vi "WPI_CANTalonSRX_Global.vi"(4 "32-bit Frame":u32, 6 "Set Boolean":bool, 7 "Write After Receive":T2, 8 "Set Number":dbl, 9 "Control Mode":T1, 10 "Operation":T7, 11 "Device ID (0)":u8) -> (1 "Get All":T2, 3 "Device ID Out":u8, 5 "Read For Send":T3={"Output"=0.0, "Control Mode"=enum."Percent VBus", "Brake-Mode Override"=enum."No Override", "Reverse Feedback Sensor"=FALSE, "Reverse Closed-Loop Output"=FALSE, "Override Limits"=FALSE, "Forward Limit Enabled"=FALSE, "Reverse Limit Enabled"=FALSE, "Feedback Select"=0, "Profile Select"=0, "Master To Follow"=0, "Throttle Ramp Rate"=0, "Disabled"=FALSE, "Encoder Codes Per Rev"=0, "Num Pot Turns"=0, "Control Frame Rate Ms"=0, "Use Control5 If Supported"=FALSE, "Enable Frame Rate Ms"=10, "Motion Profile Flow Control"=0, "Motion Profile Control Frame Rate"=10, "Talon SRX Motion Profile Trajectory Point"={"Duration Ms"=0, "Velocity"=0.0, "Position"=0.0, "Profile Slot Select"=0, "Is Last"=FALSE, "Velocity Only"=FALSE, "Zero Position"=FALSE, "Compress Code"=0, "Same Velocity"=0, "Delta Position"=0, "Count"=0}, "Current Limit Enabled"=FALSE} {"Feedback Select" items=["Digital Quadrature Encoder"=0, "Analog Pot"=2, "Analog Encoder"=3, "Count on Quad-A (Rising-Edge)"=4, "Count on Quad-A (Falling-Edge)"=5, "Position is Pulse-Width"=8, "CTR Magnetic Enc (Relative)"=6, "CTR Magnetic Enc (Absolute)"=7]})   [LabVIEW 2016]
uses:
  <vilib>/Rock Robotics/WPI/ThirdParty/CanMotor/TalonSRX/WPI_CANTalonSRX_GlobalOps.ctl
  <vilib>/Rock Robotics/WPI/ThirdParty/CanMotor/TalonSRX/WPI_CANTalonSRX_GlobalControl.ctl
  <vilib>/Rock Robotics/WPI/ThirdParty/CanMotor/TalonSRX/WPI_CANTalonSRX_APIControlMode.ctl
  <vilib>/Rock Robotics/WPI/ThirdParty/CanMotor/TalonSRX/WPI_CANTalonSRX_BrakeOverride.ctl
  <vilib>/Rock Robotics/WPI/ThirdParty/CanMotor/TalonSRX/WPI_CANTalonSRX_FeedbackSelect.ctl
  <vilib>/Rock Robotics/WPI/ThirdParty/CanMotor/TalonSRX/WPI_CANTalonSRX_MotionProfileTrajectoryPt.ctl
  <vilib>/Rock Robotics/WPI/ThirdParty/CanMotor/TalonSRX/WPI_CANTalonSRX_GlobalStatus.ctl
  <vilib>/Rock Robotics/WPI/ThirdParty/CanMotor/TalonSRX/WPI_CANTalonSRX_MessageIDs.ctl
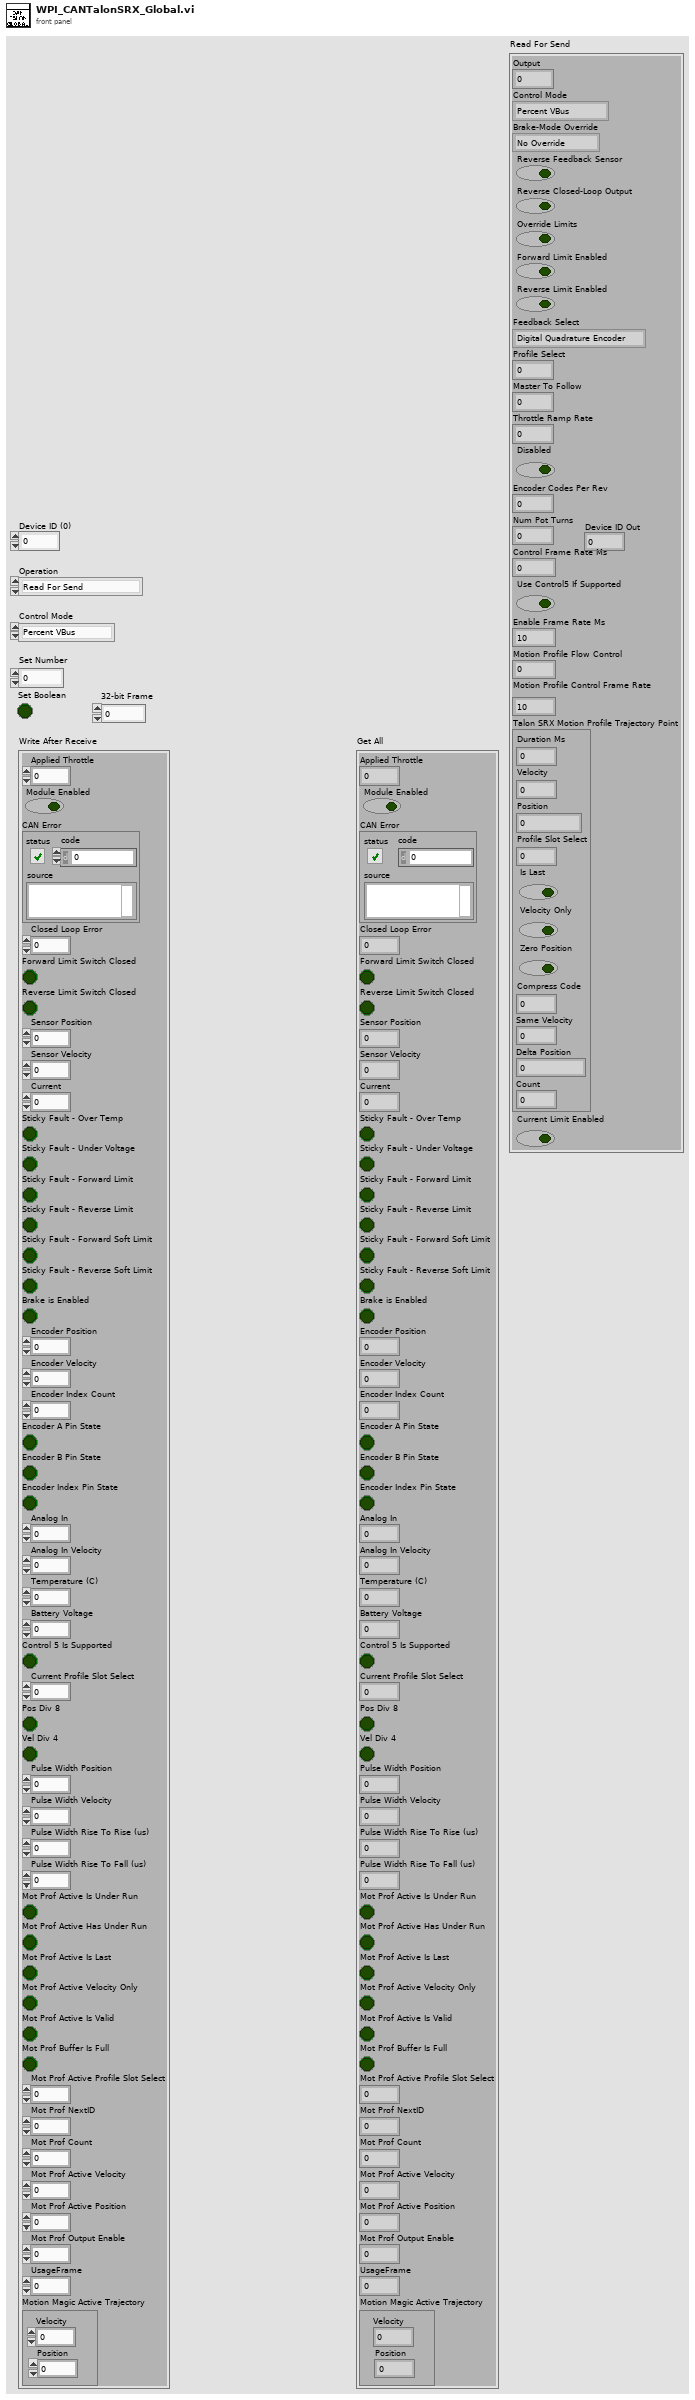
[diagram p1: front panel]
types:
  T1 = typedef "WPI_CANTalonSRX_APIControlMode.ctl" = enum8{"Percent VBus", "Speed", "Position", "Slave", "Unchanged / Invalid", "Voltage Compensation", "Current", "Motion Profile", "Motion Magic"}
  T2 = typedef "WPI_CANTalonSRX_GlobalStatus.ctl" = cluster{"Applied Throttle":dbl, "Module Enabled":bool, "CAN Error":errorcluster, "Closed Loop Error":dbl, "Forward Limit Switch Closed":bool, "Reverse Limit Switch Closed":bool, "Sensor Position":dbl, "Sensor Velocity":dbl, "Current":dbl, "Sticky Fault - Over Temp":bool, "Sticky Fault - Under Voltage":bool, "Sticky Fault - Forward Limit":bool, "Sticky Fault - Reverse Limit":bool, "Sticky Fault - Forward Soft Limit":bool, "Sticky Fault - Reverse Soft Limit":bool, "Brake is Enabled":bool, "Encoder Position":dbl, "Encoder Velocity":dbl, "Encoder Index Count":dbl, "Encoder A Pin State":bool, "Encoder B Pin State":bool, "Encoder Index Pin State":bool, "Analog In":dbl, "Analog In Velocity":dbl, "Temperature (C)":dbl, "Battery Voltage":dbl, "Control 5 Is Supported":bool, "Current Profile Slot Select":dbl, "Pos Div 8":bool, "Vel Div 4":bool, "Pulse Width Position":i32, "Pulse Width Velocity":i32, "Pulse Width Rise To Rise (us)":i32, "Pulse Width Rise To Fall (us)":i32, "Mot Prof Active Is Under Run":bool, "Mot Prof Active Has Under Run":bool, "Mot Prof Active Is Last":bool, "Mot Prof Active Velocity Only":bool, "Mot Prof Active Is Valid":bool, "Mot Prof Buffer Is Full":bool, "Mot Prof Active Profile Slot Select":i32, "Mot Prof NextID":i32, "Mot Prof Count":i32, "Mot Prof Active Velocity":dbl, "Mot Prof Active Position":dbl, "Mot Prof Output Enable":i32, "UsageFrame":u32, "Motion Magic Active Trajectory":cluster{"Velocity":dbl, "Position":dbl}}
  T3 = typedef "WPI_CANTalonSRX_GlobalControl.ctl" = cluster{"Output":dbl, "Control Mode":T1, "Brake-Mode Override":T4, "Reverse Feedback Sensor":bool, "Reverse Closed-Loop Output":bool, "Override Limits":bool, "Forward Limit Enabled":bool, "Reverse Limit Enabled":bool, "Feedback Select":T5, "Profile Select":u8, "Master To Follow":u8, "Throttle Ramp Rate":u8, "Disabled":bool, "Encoder Codes Per Rev":u32, "Num Pot Turns":u32, "Control Frame Rate Ms":u8, "Use Control5 If Supported":bool, "Enable Frame Rate Ms":u8, "Motion Profile Flow Control":u8, "Motion Profile Control Frame Rate":u8, "Talon SRX Motion Profile Trajectory Point":T6, "Current Limit Enabled":bool}
  T4 = typedef "WPI_CANTalonSRX_BrakeOverride.ctl" = enum8{"No Override", "Override to Coast", "Override to Brake"}
  T5 = typedef "WPI_CANTalonSRX_FeedbackSelect.ctl" = u8
  T6 = typedef "WPI_CANTalonSRX_MotionProfileTrajectoryPt.ctl" = cluster{"Duration Ms":u8, "Velocity":dbl, "Position":dbl, "Profile Slot Select":u8, "Is Last":bool, "Velocity Only":bool, "Zero Position":bool, "Compress Code":u8, "Same Velocity":i32, "Delta Position":i32, "Count":u8}
  T7 = typedef "WPI_CANTalonSRX_GlobalOps.ctl" = enum16{"Read For Send", "Write After Receive General", "Write After Receive Feedback", "Write After Receive Encoder", "Write After Receive Ain", "Write Error", "Get All", "Set Output", "Set Mode", "Set Master ID", "Set Brake Mode", "Set Reverse Feedback Sensor", "Set Reverse Closed Loop Output", "Set Override Limits", "Set Forward Limit Enabled", "Set Reverse Limit Enabled", "Set Feedback Select", "Set Profile Select", "Set Throttle Ramp Rate", "Disable", "Set Enc Codes Per Rev", "Set Num Pot Turns", "Set Control Frame Rate", "Enable Legacy Control", "Write After Receive Pulse Width", "Set Enable Frame Rate", "Write After Receive Motion Profile", "Set Motion Profile Flow Control", "Set Motion Profile Control Frame Rate", "Set Current Limit Enable", "Set Usage Frame", "Write After Receive Motion Magic"}
  T8 = typedef "WPI_CANTalonSRX_MessageIDs.ctl" = u32
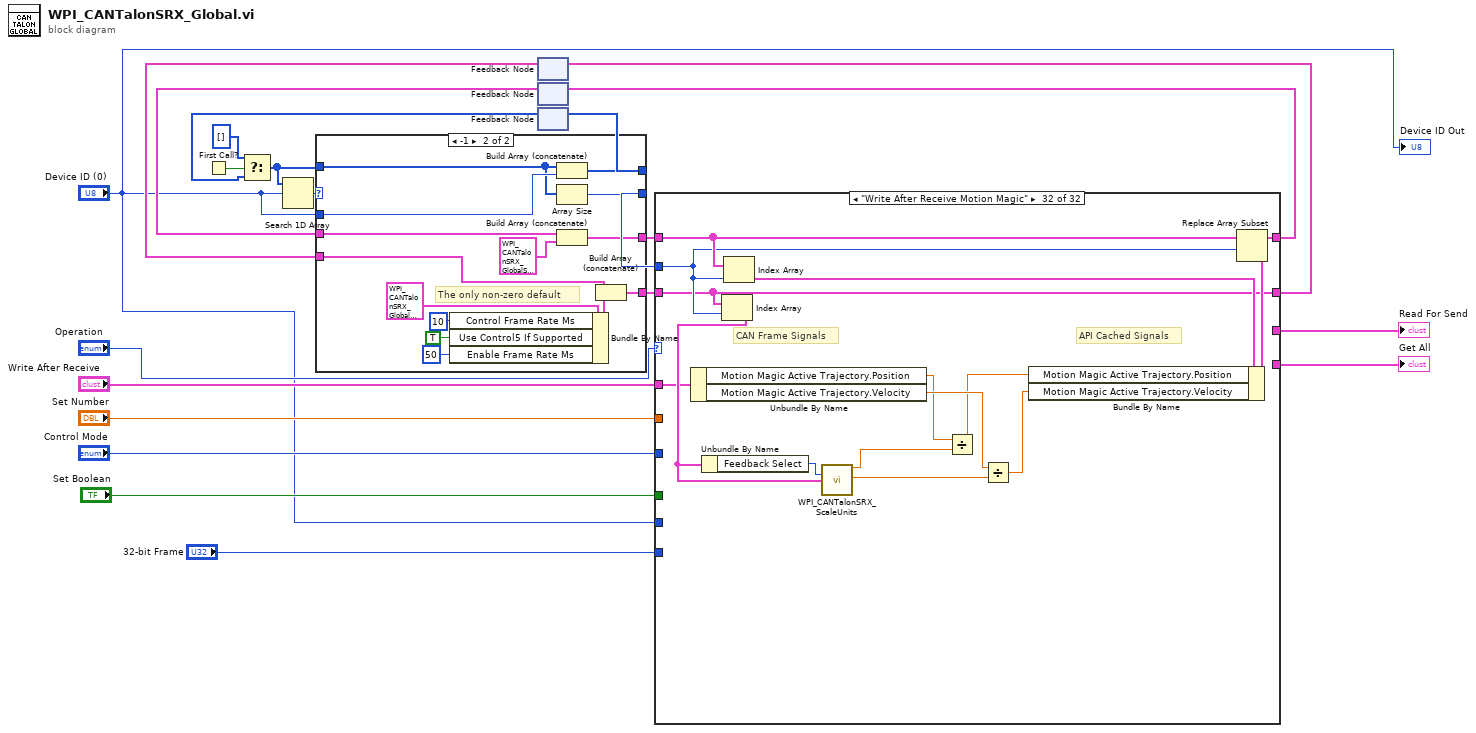
[diagram p0: block diagram]
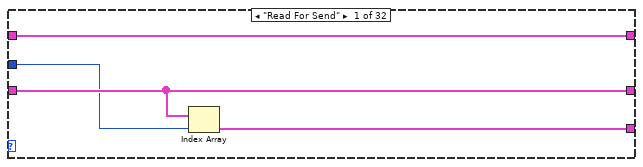
[diagram p2: hidden frame]
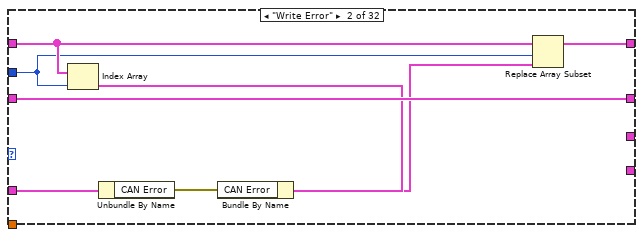
[diagram p3: hidden frame]
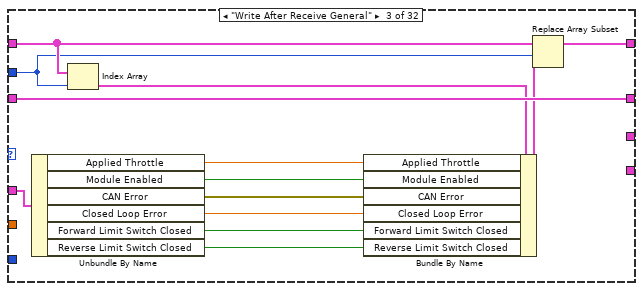
[diagram p4: hidden frame]
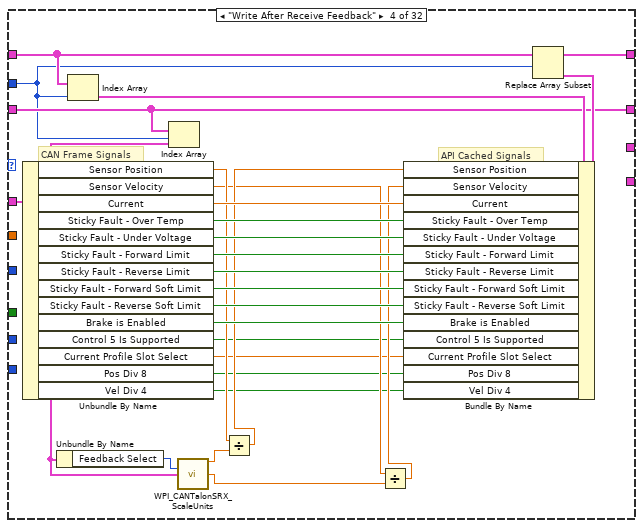
[diagram p5: hidden frame]
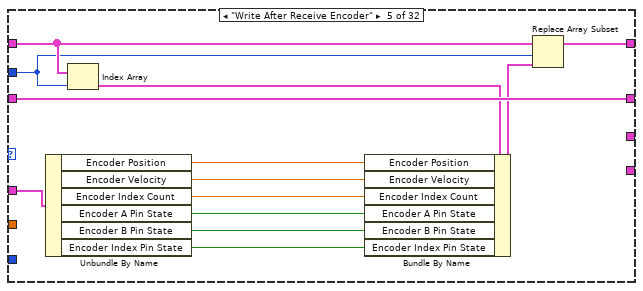
[diagram p6: hidden frame]
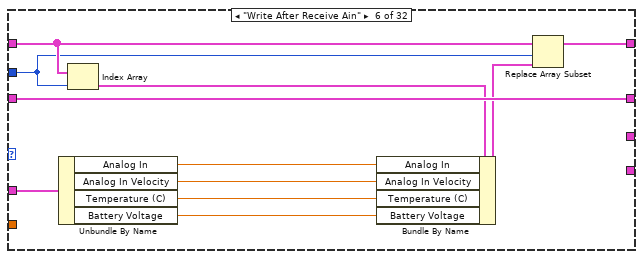
[diagram p7: hidden frame]
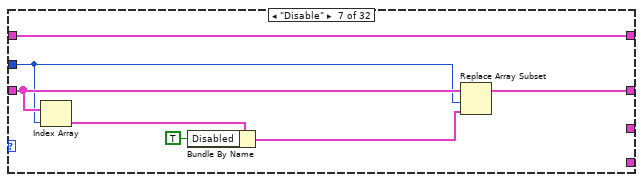
[diagram p8: hidden frame]
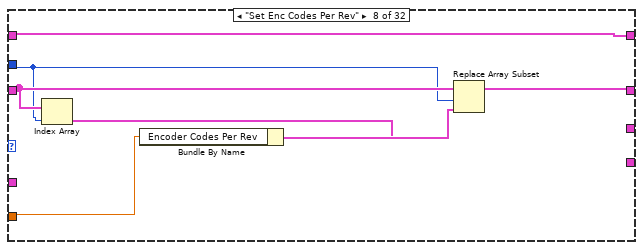
[diagram p9: hidden frame]
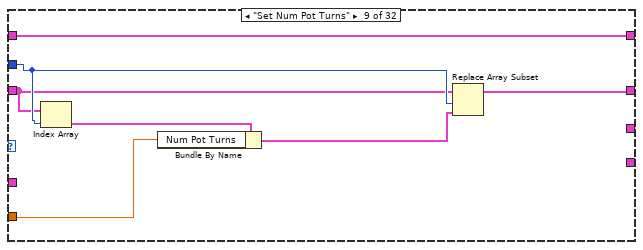
[diagram p10: hidden frame]
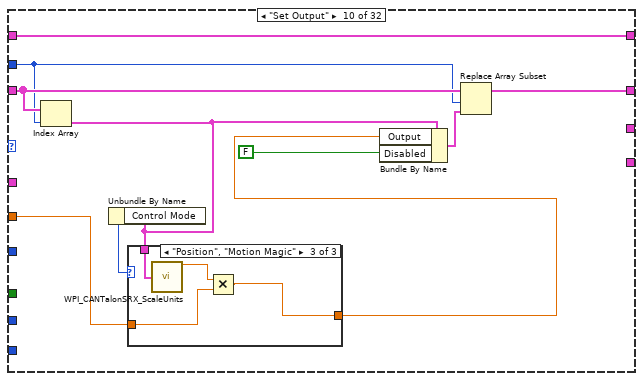
[diagram p11: hidden frame]
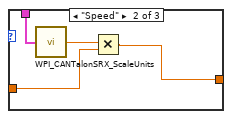
[diagram p13: hidden frame]
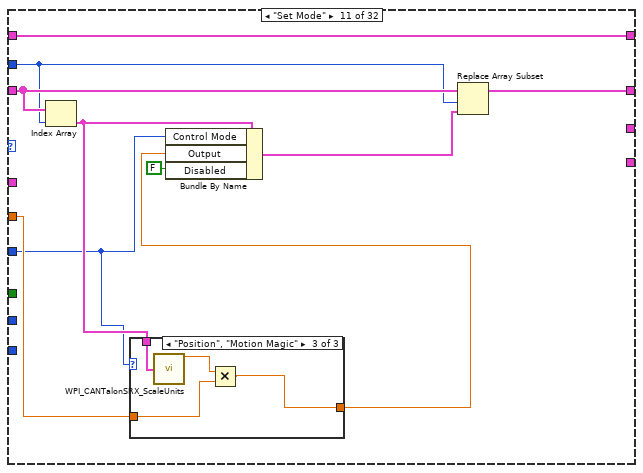
[diagram p14: hidden frame]
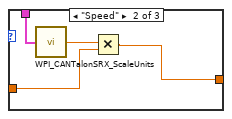
[diagram p16: hidden frame]
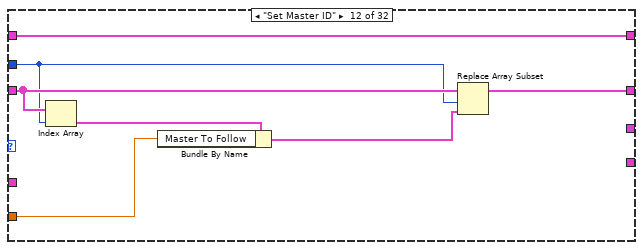
[diagram p17: hidden frame]
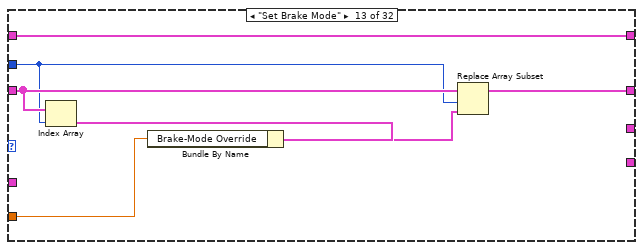
[diagram p18: hidden frame]
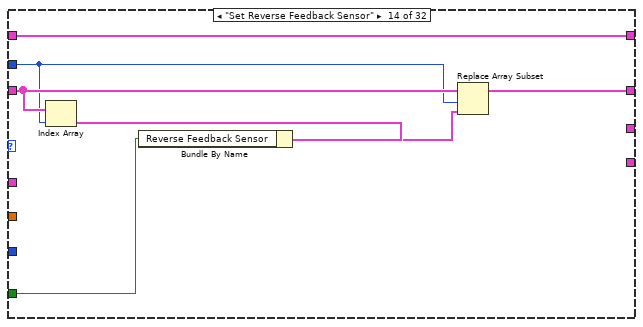
[diagram p19: hidden frame]
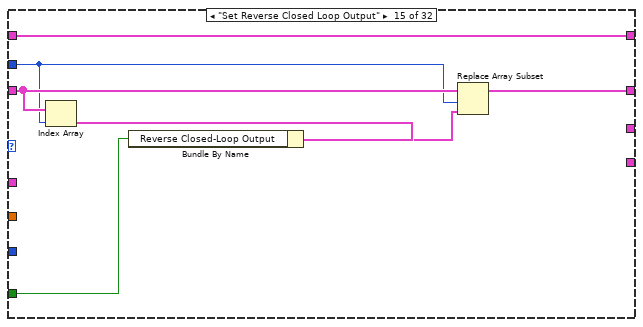
[diagram p20: hidden frame]
diagram:
  n1 = First Call?() -> (First Call?: T/F=w22:bool)
  n2 = feedback #1() -> (w15:T3[])  [unwired: 1 in]
  n3 = feedback #2() -> (w16:T2[])  [unwired: 1 in]
  n4 = feedback #3() -> (w20:u8[])  [unwired: 1 in]
  n5 = Select(t=u8[] [], s=w22, f=w20) -> (s? t:f=w18:u8[])
  n6 = Search 1D Array(1D array=w18, element="Device ID (0)") -> (index of element=w17:i32)  [unwired: 1 in]
  n7 = case shown="-1" w17 {
    selector: w17 -> [w23 _]
    tunnel: [w26 w40] -> w19
    tunnel: "Device ID (0)" -> [_ w39]
    tunnel: w18 -> [w26 w34]
    tunnel: w16 -> [w25 w38]
    tunnel: w15 -> [w24 w37]
    tunnel: [w25 w36] -> w13
    tunnel: [w24 w35] -> w11
    tunnel: [w23 w33] -> w10
    frame Default {
    }
    frame -1 {
      # "The only non-zero default"
      n8 = Bundle By Name(cluster=T3 {"Output"=0.0, "Control Mode"=enum."Percent VBus", "Brake-Mode Override"=enum."No Override", "Reverse Feedback Sensor"=FALSE, "Reverse Closed-Loop Output"=FALSE, "Override Limits"=FALSE, "Forward Limit Enabled"=FALSE, "Reverse Limit Enabled"=FALSE, "Feedback Select"=0, "Profile Select"=0, "Master To Follow"=0, "Throttle Ramp Rate"=0, "Disabled"=FALSE, "Encoder Codes Per Rev"=0, "Num Pot Turns"=0, "Control Frame Rate Ms"=0, "Use Control5 If Supported"=FALSE, "Enable Frame Rate Ms"=10, "Motion Profile Flow Control"=0, "Motion Profile Control Frame Rate"=10, "Talon SRX Motion Profile Trajectory Point"={"Duration Ms"=0, "Velocity"=0.0, "Position"=0.0, "Profile Slot Select"=0, "Is Last"=FALSE, "Velocity Only"=FALSE, "Zero Position"=FALSE, "Compress Code"=0, "Same Velocity"=0, "Delta Position"=0, "Count"=0}, "Current Limit Enabled"=FALSE} ("Read For Send"), "Control Frame Rate Ms"=u8 10, "Use Control5 If Supported"=TRUE, "Enable Frame Rate Ms"=u8 50) -> (w31:T3)
      n9 = Build Array (concatenate)(w34, w39) -> (w40:u8[])
      n10 = Array Size(array=w34) -> (size(s)=w33:i32)
      n11 = Build Array (concatenate)(w38, T2 {"Applied Throttle"=0.0, "Module Enabled"=FALSE, "CAN Error"={"status"=FALSE, "code"=0, "source"=""}, "Closed Loop Error"=0.0, "Forward Limit Switch Closed"=FALSE, "Reverse Limit Switch Closed"=FALSE, "Sensor Position"=0.0, "Sensor Velocity"=0.0, "Current"=0.0, "Sticky Fault - Over Temp"=FALSE, "Sticky Fault - Under Voltage"=FALSE, "Sticky Fault - Forward Limit"=FALSE, "Sticky Fault - Reverse Limit"=FALSE, "Sticky Fault - Forward Soft Limit"=FALSE, "Sticky Fault - Reverse Soft Limit"=FALSE, "Brake is Enabled"=FALSE, "Encoder Position"=0.0, "Encoder Velocity"=0.0, "Encoder Index Count"=0.0, "Encoder A Pin State"=FALSE, "Encoder B Pin State"=FALSE, "Encoder Index Pin State"=FALSE, "Analog In"=0.0, "Analog In Velocity"=0.0, "Temperature (C)"=0.0, "Battery Voltage"=0.0, "Control 5 Is Supported"=FALSE, "Current Profile Slot Select"=0.0, "Pos Div 8"=FALSE, "Vel Div 4"=FALSE, "Pulse Width Position"=0, "Pulse Width Velocity"=0, "Pulse Width Rise To Rise (us)"=0, "Pulse Width Rise To Fall (us)"=0, "Mot Prof Active Is Under Run"=FALSE, "Mot Prof Active Has Under Run"=FALSE, "Mot Prof Active Is Last"=FALSE, "Mot Prof Active Velocity Only"=FALSE, "Mot Prof Active Is Valid"=FALSE, "Mot Prof Buffer Is Full"=FALSE, "Mot Prof Active Profile Slot Select"=0, "Mot Prof NextID"=0, "Mot Prof Count"=0, "Mot Prof Active Velocity"=0.0, "Mot Prof Active Position"=0.0, "Mot Prof Output Enable"=0, "UsageFrame"=0, "Motion Magic Active Trajectory"={"Velocity"=0.0, "Position"=0.0}} ("Write After Receive")) -> (w36:T2[])
      n12 = Build Array (concatenate)(w37, w31) -> (w35:T3[])
    }
  }
  n13 = feedback-in #3(w19) -> ()
  n14 = case shown="\"Write After Receive Motion Magic\"" "Operation" {
    tunnel: [w44 w51 w64 w92 w104 w115 w123 w129 w131 w147 w162 w177 w184 w191 w198 w205 w212 w219 w226 w233 w240 w247 w253 w265 w274 w284 w307 w321 w325 w336 w343 w352] -> w14
    tunnel: w13 -> [w44 w50 w63 w91 w103 w114 w123 w129 w131 w147 w162 w177 w184 w191 w198 w205 w212 w219 w226 w233 w240 w247 w253 w265 w275 w284 w308 w321 w325 w336 w342 w355]
    tunnel: [w43 w52 w65 w79 w105 w116 w121 w126 w134 w145 w166 w182 w189 w196 w203 w210 w217 w224 w231 w238 w245 w249 w255 w262 w273 w283 w297 w320 w324 w333 w340 w353] -> w12
    tunnel: w11 -> [w43 w52 w65 w79 w105 w116 w122 w128 w132 w146 w165 w181 w188 w195 w202 w209 w216 w223 w230 w237 w244 w249 w256 w263 w273 w285 w297 w318 w327 w334 w340 w353]
    tunnel: w10 -> [w42 w49 w62 w78 w102 w113 w120 w125 w133 w144 w164 w180 w187 w194 w201 w208 w215 w222 w229 w236 w243 w248 w254 w264 w276 w286 w296 w322 w326 w335 w341 w354]
    tunnel: [w41 _ _ _ _ _ _ _ _ _ _ _ _ _ _ _ _ _ _ _ _ _ _ _ _ _ _ _ _ _ _ _] -> w9
    tunnel: "Write After Receive" -> [_ w46 w61 w90 w101 w112 _ _ _ _ _ _ _ _ _ _ _ _ _ _ _ _ _ _ w272 _ w309 _ _ _ _ w350]
    tunnel: "Set Number" -> [_ _ _ _ _ _ _ w127 w135 w140 w160 w176 w183 _ _ _ _ _ w225 w232 w239 _ w251 _ _ w287 _ w317 w328 _ _ _]
    tunnel: [_ _ _ _ _ _ _ _ _ _ _ _ _ _ _ _ _ _ _ _ _ w246 _ _ _ _ _ _ _ _ _ _] -> w6
    tunnel: "Control Mode" -> [_ _ _ _ _ _ _ _ _ _ w157 _ _ _ _ _ _ _ _ _ _ _ _ _ _ _ _ _ _ _ _ _]
    tunnel: "Set Boolean" -> [_ _ _ _ _ _ _ _ _ _ _ _ _ w190 w197 w204 w211 w218 _ _ _ _ _ w259 _ _ _ _ _ w332 _ _]
    tunnel: "Device ID (0)" -> [_ _ _ _ _ _ _ _ _ _ _ _ _ _ _ _ _ _ _ _ _ _ _ w260 _ _ _ _ _ _ _ _]
    tunnel: "32-bit Frame" -> [_ _ _ _ _ _ _ _ _ _ _ _ _ _ _ _ _ _ _ _ _ _ _ _ _ _ _ _ _ _ w339 _]
    frame "Read For Send" {
      n15 = Index Array(array=w43, index=w42) -> (element=w41:T3)
    }
    frame "Write Error" {
      n16 = Index Array(array=w50, index=w49) -> (element=w48:T2)
      n17 = Unbundle By Name(w46) -> ("CAN Error"=w45:errorcluster)
      n18 = Bundle By Name(cluster=w48, "CAN Error"=w45) -> (w47:T2)
      n19 = Replace Array Subset(array=w50, new element=w47, index=w49) -> (w51:T2[])
    }
    frame "Write After Receive General" {
      n20 = Unbundle By Name(w61) -> ("Applied Throttle"=w58:dbl, "Module Enabled"=w57:bool, "CAN Error"=w56:errorcluster, "Closed Loop Error"=w55:dbl, "Forward Limit Switch Closed"=w54:bool, "Reverse Limit Switch Closed"=w53:bool)
      n21 = Index Array(array=w63, index=w62) -> (element=w60:T2)
      n22 = Bundle By Name(cluster=w60, "Applied Throttle"=w58, "Module Enabled"=w57, "CAN Error"=w56, "Closed Loop Error"=w55, "Forward Limit Switch Closed"=w54, "Reverse Limit Switch Closed"=w53) -> (w59:T2)
      n23 = Replace Array Subset(array=w63, new element=w59, index=w62) -> (w64:T2[])
    }
    frame "Write After Receive Feedback" {
      # "API Cached Signals"
      # "CAN Frame Signals"
      n24 = Unbundle By Name(w90) -> ("Sensor Position"=w76:dbl, "Sensor Velocity"=w74:dbl, "Current"=w87:dbl, "Sticky Fault - Over Temp"=w86:bool, "Sticky Fault - Under Voltage"=w85:bool, "Sticky Fault - Forward Limit"=w84:bool, "Sticky Fault - Reverse Limit"=w80:bool, "Sticky Fault - Forward Soft Limit"=w81:bool, "Sticky Fault - Reverse Soft Limit"=w82:bool, "Brake is Enabled"=w83:bool, "Control 5 Is Supported"=w66:bool, "Current Profile Slot Select"=w67:dbl, "Pos Div 8"=w68:bool, "Vel Div 4"=w69:bool)
      n25 = Index Array(array=w91, index=w78) -> (element=w89:T2)
      n26 = Index Array(array=w79, index=w78) -> (element=w71:T3)
      n27 = Unbundle By Name(w71) -> ("Feedback Select"=w70:T5)
      n28 = call <vilib>:"WPI_CANTalonSRX_ScaleUnits.vi"("Feedback Scalar Select"=w70, "Read For Send"=w71) -> ("Position Scalar"=w75:dbl, "Velocity Scalar"=w73:dbl)  [unwired: 11 in, 1 out]
      n29 = Divide(x=w76, y=w75) -> (x/y=w77:dbl)
      n30 = Divide(x=w74, y=w73) -> (x/y=w72:dbl)
      n31 = Bundle By Name(cluster=w89, "Sensor Position"=w77, "Sensor Velocity"=w72, "Current"=w87, "Sticky Fault - Over Temp"=w86, "Sticky Fault - Under Voltage"=w85, "Sticky Fault - Forward Limit"=w84, "Sticky Fault - Reverse Limit"=w80, "Sticky Fault - Forward Soft Limit"=w81, "Sticky Fault - Reverse Soft Limit"=w82, "Brake is Enabled"=w83, "Control 5 Is Supported"=w66, "Current Profile Slot Select"=w67, "Pos Div 8"=w68, "Vel Div 4"=w69) -> (w88:T2)
      n32 = Replace Array Subset(array=w91, new element=w88, index=w78) -> (w92:T2[])
    }
    frame "Write After Receive Encoder" {
      n33 = Unbundle By Name(w101) -> ("Encoder Position"=w98:dbl, "Encoder Velocity"=w97:dbl, "Encoder Index Count"=w96:dbl, "Encoder A Pin State"=w95:bool, "Encoder B Pin State"=w94:bool, "Encoder Index Pin State"=w93:bool)
      n34 = Index Array(array=w103, index=w102) -> (element=w100:T2)
      n35 = Bundle By Name(cluster=w100, "Encoder Position"=w98, "Encoder Velocity"=w97, "Encoder Index Count"=w96, "Encoder A Pin State"=w95, "Encoder B Pin State"=w94, "Encoder Index Pin State"=w93) -> (w99:T2)
      n36 = Replace Array Subset(array=w103, new element=w99, index=w102) -> (w104:T2[])
    }
    frame "Write After Receive Ain" {
      n37 = Unbundle By Name(w112) -> ("Analog In"=w109:dbl, "Analog In Velocity"=w108:dbl, "Temperature (C)"=w107:dbl, "Battery Voltage"=w106:dbl)
      n38 = Index Array(array=w114, index=w113) -> (element=w111:T2)
      n39 = Bundle By Name(cluster=w111, "Analog In"=w109, "Analog In Velocity"=w108, "Temperature (C)"=w107, "Battery Voltage"=w106) -> (w110:T2)
      n40 = Replace Array Subset(array=w114, new element=w110, index=w113) -> (w115:T2[])
    }
    frame "Disable" {
      n41 = Index Array(array=w122, index=w120) -> (element=w119:T3)
      n42 = Bundle By Name(cluster=w119, "Disabled"=TRUE) -> (w118:T3)
      n43 = Replace Array Subset(array=w122, new element=w118, index=w120) -> (w121:T3[])
    }
    frame "Set Enc Codes Per Rev" {
      n44 = Index Array(array=w128, index=w125) -> (element=w124:T3)
      n45 = Bundle By Name(cluster=w124, "Encoder Codes Per Rev"=w127) -> (w130:T3)
      n46 = Replace Array Subset(array=w128, new element=w130, index=w125) -> (w126:T3[])
    }
    frame "Set Num Pot Turns" {
      n47 = Index Array(array=w132, index=w133) -> (element=w136:T3)
      n48 = Bundle By Name(cluster=w136, "Num Pot Turns"=w135) -> (w137:T3)
      n49 = Replace Array Subset(array=w132, new element=w137, index=w133) -> (w134:T3[])
    }
    frame "Set Output" {
      n50 = Index Array(array=w146, index=w144) -> (element=w138:T3)
      n51 = Unbundle By Name(w138) -> ("Control Mode"=w141:T1)
      n52 = case shown="\"Position\", \"Motion Magic\"" w141 {
        tunnel: [w148 w149 w155] -> w139
        tunnel: w140 -> [w148 w151 w153]
        tunnel: w138 -> [_ w152 w156]
        frame Default {
        }
        frame "Speed" {
          n53 = call <vilib>:"WPI_CANTalonSRX_ScaleUnits.vi"("Read For Send"=w152) -> ("Velocity Scalar"=w150:dbl)  [unwired: 12 in, 2 out]
          n54 = Multiply(x=w150, y=w151) -> (x*y=w149:dbl)
        }
        frame "Position", "Motion Magic" {
          n55 = call <vilib>:"WPI_CANTalonSRX_ScaleUnits.vi"("Read For Send"=w156) -> ("Position Scalar"=w154:dbl)  [unwired: 12 in, 2 out]
          n56 = Multiply(x=w154, y=w153) -> (x*y=w155:dbl)
        }
      }
      n57 = Bundle By Name(cluster=w138, "Output"=w139, "Disabled"=FALSE) -> (w143:T3)
      n58 = Replace Array Subset(array=w146, new element=w143, index=w144) -> (w145:T3[])
    }
    frame "Set Mode" {
      n59 = Index Array(array=w165, index=w164) -> (element=w158:T3)
      n60 = case shown="\"Position\", \"Motion Magic\"" w157 {
        tunnel: [w167 w168 w174] -> w159
        tunnel: w160 -> [w167 w170 w172]
        tunnel: w158 -> [_ w171 w175]
        frame Default {
        }
        frame "Speed" {
          n61 = call <vilib>:"WPI_CANTalonSRX_ScaleUnits.vi"("Read For Send"=w171) -> ("Velocity Scalar"=w169:dbl)  [unwired: 12 in, 2 out]
          n62 = Multiply(x=w169, y=w170) -> (x*y=w168:dbl)
        }
        frame "Position", "Motion Magic" {
          n63 = call <vilib>:"WPI_CANTalonSRX_ScaleUnits.vi"("Read For Send"=w175) -> ("Position Scalar"=w173:dbl)  [unwired: 12 in, 2 out]
          n64 = Multiply(x=w173, y=w172) -> (x*y=w174:dbl)
        }
      }
      n65 = Bundle By Name(cluster=w158, "Control Mode"=w157, "Output"=w159, "Disabled"=FALSE) -> (w163:T3)
      n66 = Replace Array Subset(array=w165, new element=w163, index=w164) -> (w166:T3[])
    }
    frame "Set Master ID" {
      n67 = Index Array(array=w181, index=w180) -> (element=w179:T3)
      n68 = Bundle By Name(cluster=w179, "Master To Follow"=w176) -> (w178:T3)
      n69 = Replace Array Subset(array=w181, new element=w178, index=w180) -> (w182:T3[])
    }
    frame "Set Brake Mode" {
      n70 = Index Array(array=w188, index=w187) -> (element=w186:T3)
      n71 = Bundle By Name(cluster=w186, "Brake-Mode Override"=w183) -> (w185:T3)
      n72 = Replace Array Subset(array=w188, new element=w185, index=w187) -> (w189:T3[])
    }
    frame "Set Reverse Feedback Sensor" {
      n73 = Index Array(array=w195, index=w194) -> (element=w193:T3)
      n74 = Bundle By Name(cluster=w193, "Reverse Feedback Sensor"=w190) -> (w192:T3)
      n75 = Replace Array Subset(array=w195, new element=w192, index=w194) -> (w196:T3[])
    }
    frame "Set Reverse Closed Loop Output" {
      n76 = Index Array(array=w202, index=w201) -> (element=w200:T3)
      n77 = Bundle By Name(cluster=w200, "Reverse Closed-Loop Output"=w197) -> (w199:T3)
      n78 = Replace Array Subset(array=w202, new element=w199, index=w201) -> (w203:T3[])
    }
    frame "Set Override Limits" {
      n79 = Index Array(array=w209, index=w208) -> (element=w207:T3)
      n80 = Bundle By Name(cluster=w207, "Override Limits"=w204) -> (w206:T3)
      n81 = Replace Array Subset(array=w209, new element=w206, index=w208) -> (w210:T3[])
    }
    frame "Set Forward Limit Enabled" {
      n82 = Index Array(array=w216, index=w215) -> (element=w214:T3)
      n83 = Bundle By Name(cluster=w214, "Forward Limit Enabled"=w211) -> (w213:T3)
      n84 = Replace Array Subset(array=w216, new element=w213, index=w215) -> (w217:T3[])
    }
    frame "Set Reverse Limit Enabled" {
      n85 = Index Array(array=w223, index=w222) -> (element=w221:T3)
      n86 = Bundle By Name(cluster=w221, "Reverse Limit Enabled"=w218) -> (w220:T3)
      n87 = Replace Array Subset(array=w223, new element=w220, index=w222) -> (w224:T3[])
    }
    frame "Set Feedback Select" {
      n88 = Index Array(array=w230, index=w229) -> (element=w228:T3)
      n89 = Bundle By Name(cluster=w228, "Feedback Select"=w225) -> (w227:T3)
      n90 = Replace Array Subset(array=w230, new element=w227, index=w229) -> (w231:T3[])
    }
    frame "Set Profile Select" {
      n91 = Index Array(array=w237, index=w236) -> (element=w235:T3)
      n92 = Bundle By Name(cluster=w235, "Profile Select"=w232) -> (w234:T3)
      n93 = Replace Array Subset(array=w237, new element=w234, index=w236) -> (w238:T3[])
    }
    frame "Set Throttle Ramp Rate" {
      n94 = Index Array(array=w244, index=w243) -> (element=w242:T3)
      n95 = Bundle By Name(cluster=w242, "Throttle Ramp Rate"=w239) -> (w241:T3)
      n96 = Replace Array Subset(array=w244, new element=w241, index=w243) -> (w245:T3[])
    }
    frame "Get All" {
      n97 = Index Array(array=w247, index=w248) -> (element=w246:T2)
    }
    frame "Set Control Frame Rate" {
      n98 = Index Array(array=w256, index=w254) -> (element=w252:T3)
      n99 = To Unsigned Byte Integer(number=w251) -> (unsigned 8bit integer=w250:u8)
      n100 = Bundle By Name(cluster=w252, "Control Frame Rate Ms"=w250) -> (w257:T3)
      n101 = Replace Array Subset(array=w256, new element=w257, index=w254) -> (w255:T3[])
    }
    frame "Enable Legacy Control" {
      n102 = Index Array(array=w263, index=w264) -> (element=w266:T3)
      n103 = Not(x=w259) -> (.not. x?=w261:bool)
      n104 = Bundle By Name(cluster=w266, "Use Control5 If Supported"=w261) -> (w258:T3)
      n105 = case shown="True" w259 {
        tunnel: w260 -> [_ w267]
        frame False {
        }
        frame True {
          w268 = T8 33816832 items=["TalonSRX Control General 10ms"=33816576, "TalonSRX Control Rates Slow"=33816640, "TalonSRX Control ClearFlags Slow"=33816704, "TalonSRX Status General 10ms"=33821696, "TalonSRX Status Feedback 20ms"=33821760, "TalonSRX Status Enc 100ms"=33821824, "TalonSRX Status AinTempVbat 100ms"=33821888, "TalonSRX Status Startup Once"=33821952, "TalonSRX Status Debug"=33822080, "TalonSRX Config SetGainsSlot0 A"=33823808, "TalonSRX Config SetGainsSlot0 B"=33823872, "TalonSRX Config SetGainsSlot1 A"=33823936, "TalonSRX Config SetGainsSlot1 B"=33824000, "TalonSRX Config SetSoftLimits"=33824064, "TalonSRX Config WebControl"=33824128, "TalonSRX Param Request"=33822720, "TalonSRX Param Response"=33822784, "TalonSRX Param Set"=33822848, "TalonSRX Status PulseWidth"=33822144, "TalonSRX Status Motion Profile"=33822208, "TalonSRX Control General 5"=33816832, "TalonSRX Control Motion Profile Add"=33816896] ("Talon SRX Control Frame")
          # "Turn off Control 5, Send VI will use Control 1"
          n106 = Or(x=w267, y=w268) -> (x .or. y?=w269:T8)
          n107 = call <vilib>:"NetComm_CAN_Send.vi"("Period (ms)"=0, "Data"=u8[] [] ("Token Space"), "Message ID"=w269) -> ()  [unwired: 8 in, 1 out]
        }
      }
      n108 = Replace Array Subset(array=w263, new element=w258, index=w264) -> (w262:T3[])
    }
    frame "Write After Receive Pulse Width" {
      n109 = Unbundle By Name(w272) -> ("Pulse Width Position"=w280:i32, "Pulse Width Velocity"=w279:i32, "Pulse Width Rise To Rise (us)"=w278:i32, "Pulse Width Rise To Fall (us)"=w277:i32)
      n110 = Index Array(array=w275, index=w276) -> (element=w282:T2)
      n111 = Bundle By Name(cluster=w282, "Pulse Width Position"=w280, "Pulse Width Velocity"=w279, "Pulse Width Rise To Rise (us)"=w278, "Pulse Width Rise To Fall (us)"=w277) -> (w281:T2)
      n112 = Replace Array Subset(array=w275, new element=w281, index=w276) -> (w274:T2[])
    }
    frame "Set Enable Frame Rate" {
      n113 = Index Array(array=w285, index=w286) -> (element=w289:T3)
      n114 = To Unsigned Byte Integer(number=w287) -> (unsigned 8bit integer=w288:u8)
      n115 = Bundle By Name(cluster=w289, "Enable Frame Rate Ms"=w288) -> (w290:T3)
      n116 = Replace Array Subset(array=w285, new element=w290, index=w286) -> (w283:T3[])
    }
    frame "Write After Receive Motion Profile" {
      # "API Cached Signals"
      # "CAN Frame Signals"
      n117 = Unbundle By Name(w309) -> ("Mot Prof Active Is Under Run"=w313:bool, "Mot Prof Active Has Under Run"=w312:bool, "Mot Prof Active Is Last"=w311:bool, "Mot Prof Active Velocity Only"=w310:bool, "Mot Prof Active Is Valid"=w306:bool, "Mot Prof Buffer Is Full"=w305:bool, "Mot Prof Active Profile Slot Select"=w304:i32, "Mot Prof NextID"=w303:i32, "Mot Prof Count"=w302:i32, "Mot Prof Active Velocity"=w294:dbl, "Mot Prof Active Position"=w292:dbl, "Mot Prof Output Enable"=w301:i32)
      n118 = Index Array(array=w297, index=w296) -> (element=w295:T3)
      n119 = Unbundle By Name(w295) -> ("Feedback Select"=w298:T5)
      n120 = Index Array(array=w308, index=w296) -> (element=w315:T2)
      n121 = call <vilib>:"WPI_CANTalonSRX_ScaleUnits.vi"("Feedback Scalar Select"=w298, "Read For Send"=w295) -> ("Position Scalar"=w300:dbl, "Velocity Scalar"=w299:dbl)  [unwired: 11 in, 1 out]
      n122 = Divide(x=w292, y=w300) -> (x/y=w291:dbl)
      n123 = Divide(x=w294, y=w299) -> (x/y=w293:dbl)
      n124 = Bundle By Name(cluster=w315, "Mot Prof Active Is Under Run"=w313, "Mot Prof Active Has Under Run"=w312, "Mot Prof Active Is Last"=w311, "Mot Prof Active Velocity Only"=w310, "Mot Prof Active Is Valid"=w306, "Mot Prof Buffer Is Full"=w305, "Mot Prof Active Profile Slot Select"=w304, "Mot Prof NextID"=w303, "Mot Prof Count"=w302, "Mot Prof Active Velocity"=w293, "Mot Prof Active Position"=w291, "Mot Prof Output Enable"=w301) -> (w314:T2)
      n125 = Replace Array Subset(array=w308, new element=w314, index=w296) -> (w307:T2[])
    }
    frame "Set Motion Profile Flow Control" {
      n126 = Index Array(array=w318, index=w322) -> (element=w319:T3)
      n127 = To Unsigned Byte Integer(number=w317) -> (unsigned 8bit integer=w316:u8)
      n128 = Bundle By Name(cluster=w319, "Motion Profile Flow Control"=w316) -> (w323:T3)
      n129 = Replace Array Subset(array=w318, new element=w323, index=w322) -> (w320:T3[])
    }
    frame "Set Motion Profile Control Frame Rate" {
      n130 = Index Array(array=w327, index=w326) -> (element=w330:T3)
      n131 = To Unsigned Byte Integer(number=w328) -> (unsigned 8bit integer=w329:u8)
      n132 = Bundle By Name(cluster=w330, "Motion Profile Control Frame Rate"=w329) -> (w331:T3)
      n133 = Replace Array Subset(array=w327, new element=w331, index=w326) -> (w324:T3[])
    }
    frame "Set Current Limit Enable" {
      n134 = Index Array(array=w334, index=w335) -> (element=w338:T3)
      n135 = Bundle By Name(cluster=w338, "Current Limit Enabled"=w332) -> (w337:T3)
      n136 = Replace Array Subset(array=w334, new element=w337, index=w335) -> (w333:T3[])
    }
    frame "Set Usage Frame" {
      n137 = Index Array(array=w342, index=w341) -> (element=w344:T2)
      n138 = Bundle By Name(cluster=w344, "UsageFrame"=w339) -> (w345:T2)
      n139 = Replace Array Subset(array=w342, new element=w345, index=w341) -> (w343:T2[])
    }
    frame "Write After Receive Motion Magic" {
      # "API Cached Signals"
      # "CAN Frame Signals"
      n140 = Unbundle By Name(w350) -> ("Motion Magic Active Trajectory.Position"=w348:dbl, "Motion Magic Active Trajectory.Velocity"=w349:dbl)
      n141 = Index Array(array=w353, index=w354) -> (element=w351:T3)
      n142 = Unbundle By Name(w351) -> ("Feedback Select"=w360:T5)
      n143 = Index Array(array=w355, index=w354) -> (element=w356:T2)
      n144 = call <vilib>:"WPI_CANTalonSRX_ScaleUnits.vi"("Feedback Scalar Select"=w360, "Read For Send"=w351) -> ("Position Scalar"=w358:dbl, "Velocity Scalar"=w359:dbl)  [unwired: 11 in, 1 out]
      n145 = Divide(x=w348, y=w358) -> (x/y=w347:dbl)
      n146 = Divide(x=w349, y=w359) -> (x/y=w346:dbl)
      n147 = Bundle By Name(cluster=w356, "Motion Magic Active Trajectory.Position"=w347, "Motion Magic Active Trajectory.Velocity"=w346) -> (w357:T2)
      n148 = Replace Array Subset(array=w355, new element=w357, index=w354) -> (w352:T2[])
    }
  }
  "Read For Send" <- w9
  "Get All" <- w6
  n149 = feedback-in #1(w12) -> ()
  n150 = feedback-in #2(w14) -> ()
  "Device ID Out" <- "Device ID (0)"
